vi "server.Parse Response for Result or Error.vi"(8 "error in":errorcluster, 10 "Response String In":string) -> (0 "error out":errorcluster, 1 "LabVIEW Error?":bool=TRUE, 2 "JSON Value out":refnum<class "JSON Value.lvclass">)   [LabVIEW 2016, in "JSONRPC Server.lvclass"]
uses:
  JSONRPC Server.lvclass
  <vilib>/NI/JSON Support for LabVIEW/JSON Value/JSON Value.lvclass
  <vilib>/NI/JSON Support for LabVIEW/JSON Value/Parse/Parse Value.vi
  <vilib>/NI/JSON Support for LabVIEW/JSON Value/Object/Get Value/Get Value (Value).vi
  <vilib>/NI/JSON Support for LabVIEW/JSON Value/Object/Get Value/Get Value (Numeric).vi
  <vilib>/NI/JSON Support for LabVIEW/JSON Value/Object/Get Value/Get Value (String).vi
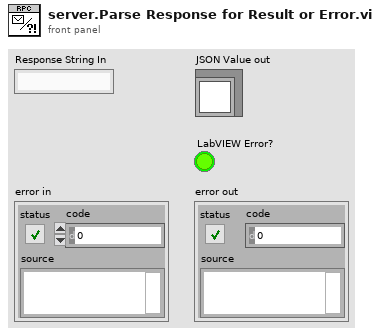
[diagram p1: front panel]
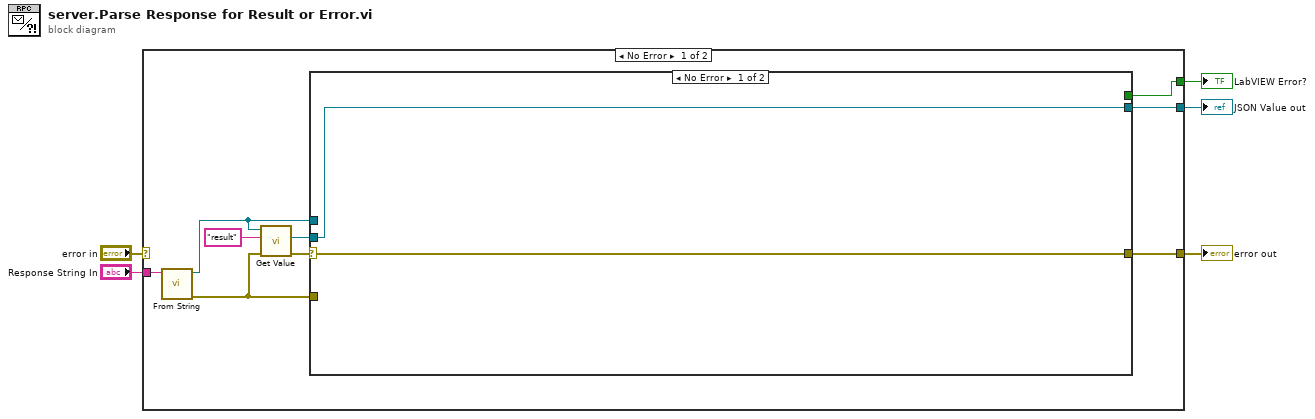
[diagram p0: block diagram]
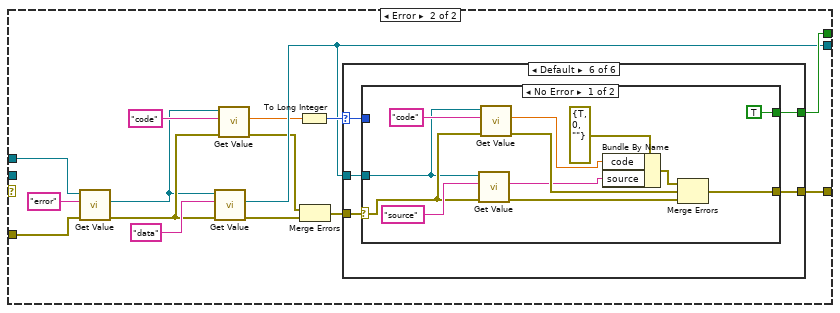
[diagram p2: hidden frame]
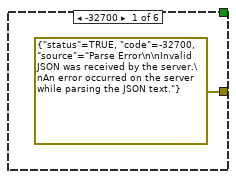
[diagram p3: hidden frame]
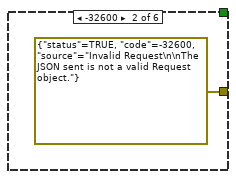
[diagram p4: hidden frame]
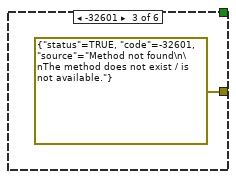
[diagram p5: hidden frame]
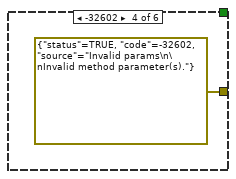
[diagram p6: hidden frame]
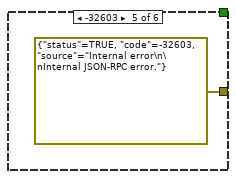
[diagram p7: hidden frame]
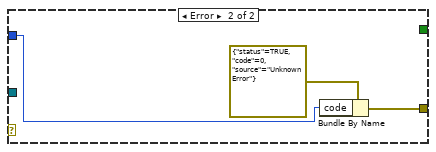
[diagram p8: hidden frame]
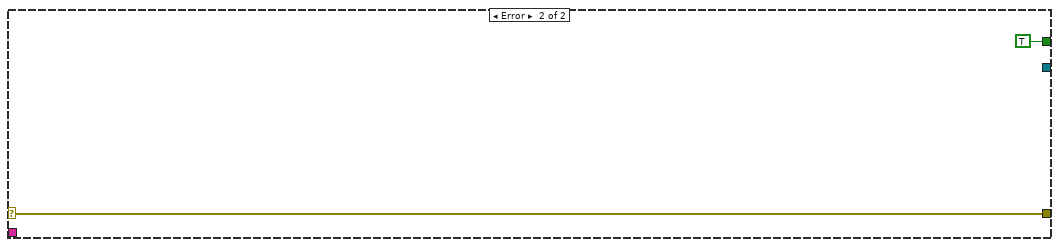
[diagram p9: hidden frame]
diagram:
  n1 = case shown="No Error" "error in" {
    selector: "error in" -> [_ w57]
    tunnel: "Response String In" -> [w11 _]
    tunnel: [w14 _] -> w1
    tunnel: [w13 w57] -> w3
    tunnel: [w12 TRUE] -> w2
    frame No Error {
      n2 = call <vilib>:"From String.vi"("JSON String"=w11) -> ("error out"=w7:errorcluster, "JSON Value out"=w6:refnum<class "JSON Value.lvclass">)  [unwired: 9 in]
      n3 = call-poly <vilib>:"Get Value.vi"("error in (no error)"=w7, "key"="result", "JSON Value in"=w6) -> ("error out"=w8:errorcluster, "JSON Value out"=w9:refnum<class "JSON Value.lvclass">)  [unwired: 7 in]
      n4 = case shown="No Error" w8 {
        selector: w8 -> [w15 _]
        tunnel: [w16 w24] -> w14
        tunnel: [w15 w30] -> w13
        tunnel: [_ w29] -> w12
        tunnel: w6 -> [_ w28]
        tunnel: w9 -> [w16 _]
        tunnel: w7 -> [_ w17]
        frame No Error {
        }
        frame Error {
          n5 = call-poly <vilib>:"Get Value.vi"("error in (no error)"=w17, "key"="error", "JSON Value in"=w28) -> ("error out"=w22:errorcluster, "JSON Value out"=w19:refnum<class "JSON Value.lvclass">)  [unwired: 7 in]
          n6 = call-poly <vilib>:"Get Value.vi"("error in (no error)"=w22, "key"="data", "JSON Value in"=w19) -> ("error out"=w21:errorcluster, "JSON Value out"=w24:refnum<class "JSON Value.lvclass">)  [unwired: 7 in]
          n7 = call-poly <vilib>:"Get Value.vi"("error in (no error)"=w22, "key"="code", "JSON Value in"=w19) -> ("error out"=w23:errorcluster, "value"=w18:dbl)  [unwired: 7 in]
          n8 = To Long Integer(number=w18) -> (32bit integer=w31:i32)
          n9 = Merge Errors(w23, w21) -> (w20:errorcluster)
          n10 = case shown="Default" w31 {
            selector: w31 -> [_ _ _ _ _ w39]
            tunnel: [errorcluster {"status"=TRUE, "code"=-32700, "source"="Parse Error\n\nInvalid JSON was received by the server.\nAn error occurred on the server while parsing the JSON text."} ("error constant") errorcluster {"status"=TRUE, "code"=-32600, "source"="Invalid Request\n\nThe JSON sent is not a valid Request object."} ("error constant") errorcluster {"status"=TRUE, "code"=-32601, "source"="Method not found\n\nThe method does not exist / is not available."} ("error constant") errorcluster {"status"=TRUE, "code"=-32602, "source"="Invalid params\n\nInvalid method parameter(s)."} ("error constant") errorcluster {"status"=TRUE, "code"=-32603, "source"="Internal error\n\nInternal JSON-RPC error."} ("error constant") w41] -> w30
            tunnel: w24 -> [_ _ _ _ _ w40]
            tunnel: [_ _ _ _ _ w38] -> w29
            tunnel: w20 -> [_ _ _ _ _ w37]
            frame -32700 {
            }
            frame -32600 {
            }
            frame -32601 {
            }
            frame -32602 {
            }
            frame -32603 {
            }
            frame Default {
              n11 = case shown="No Error" w37 {
                selector: w37 -> [w48 _]
                tunnel: [w46 w54] -> w41
                tunnel: w40 -> [w42 _]
                tunnel: w39 -> [_ w55]
                tunnel: [TRUE _] -> w38
                frame No Error {
                  n12 = call-poly <vilib>:"Get Value.vi"("error in (no error)"=w48, "key"="source" ("Parameter Name"), "JSON Value in"=w42) -> ("error out"=w49:errorcluster, "value"=w43:string)  [unwired: 7 in]
                  n13 = call-poly <vilib>:"Get Value.vi"("error in (no error)"=w48, "key"="code", "JSON Value in"=w42) -> ("error out"=w44:errorcluster, "value"=w45:dbl)  [unwired: 7 in]
                  n14 = Bundle By Name(cluster=errorcluster {"status"=TRUE, "code"=0, "source"=""} ("error constant"), "code"=w45, "source"=w43) -> (w47:errorcluster)
                  n15 = Merge Errors(w47, w44, w49) -> (w46:errorcluster)
                }
                frame Error {
                  n16 = Bundle By Name(cluster=errorcluster {"status"=TRUE, "code"=0, "source"="Unknown Error"} ("error constant"), "code"=w55) -> (w54:errorcluster)
                }
              }
            }
          }
        }
      }
    }
    frame Error {
    }
  }
  "error out" <- w3
  "JSON Value out" <- w1
  "LabVIEW Error?" <- w2
